vi "Power Values (Multiple Lines).vi"(0 "phase voltage spectra":T2(array[cluster]), 5 "current spectra":T2(array[cluster]), 9 "system info in":refnum<class "EP System Info.lvclass">, 11 "error in (no error)":errorcluster) -> (4 "power values":T4, 6 "3-phase power values":T3, 10 "system info out":refnum<class "EP System Info.lvclass">, 15 "error out":errorcluster)   [LabVIEW 2014, in "NI_EP_Power Quality.lvlib"]
doc: "Calculates the power values from the voltage and current spectra of different line configurations. You must manually select the polymorphic instance you want to use."
uses:
  <vilib>/addons/Electrical Power/PQ/NI_EP_Power Quality.lvlib
  <vilib>/addons/Electrical Power/PQ/Common/Classes/System Info/EP System Info.lvclass
  <vilib>/addons/Electrical Power/PQ/Common/Controls/ep_AI Data Channel.ctl
  <vilib>/addons/Electrical Power/Basic/NI_EP_Basic.lvlib
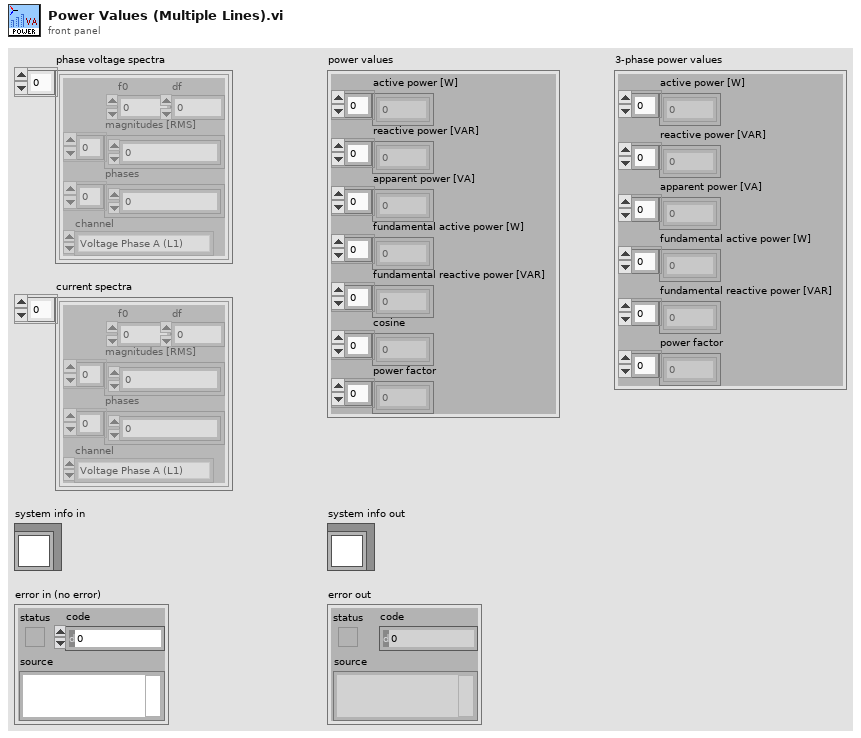
[diagram p1: front panel]
types:
  T1 = typedef "NI_EP_Power Quality.lvlib/ep_AI Data Channel.ctl" = enum16{"Voltage Phase A (L1)", "Voltage Phase B (L2)", "Voltage Phase C (L3)", "Voltage Phase N (Neutral)", "Current Phase A (L1)", "Current Phase B (L2)", "Current Phase C (L3)", "Current Phase N (Neutral)"}
  T2 = cluster{"f0":dbl, "df":dbl, "magnitudes [RMS]":dbl[], "phases":dbl[], "channel":T1}[]
  T3 = cluster{"active power [W]":dbl[], "reactive power [VAR]":dbl[], "apparent power [VA]":dbl[], "fundamental active power [W]":dbl[], "fundamental reactive power [VAR]":dbl[], "power factor":dbl[]}
  T4 = cluster{"active power [W]":dbl[], "reactive power [VAR]":dbl[], "apparent power [VA]":dbl[], "fundamental active power [W]":dbl[], "fundamental reactive power [VAR]":dbl[], "cosine":dbl[], "power factor":dbl[]}
  T5 = cluster{"active power P (W)":dbl[], "reactive power Q (VAr)":dbl[], "apparent power S (VA)":dbl[], "fundamental active power P1 (W)":dbl[], "fundamental reactive power Q1 (VAr)":dbl[], "cosine":dbl[], "power factor PF":dbl[]}
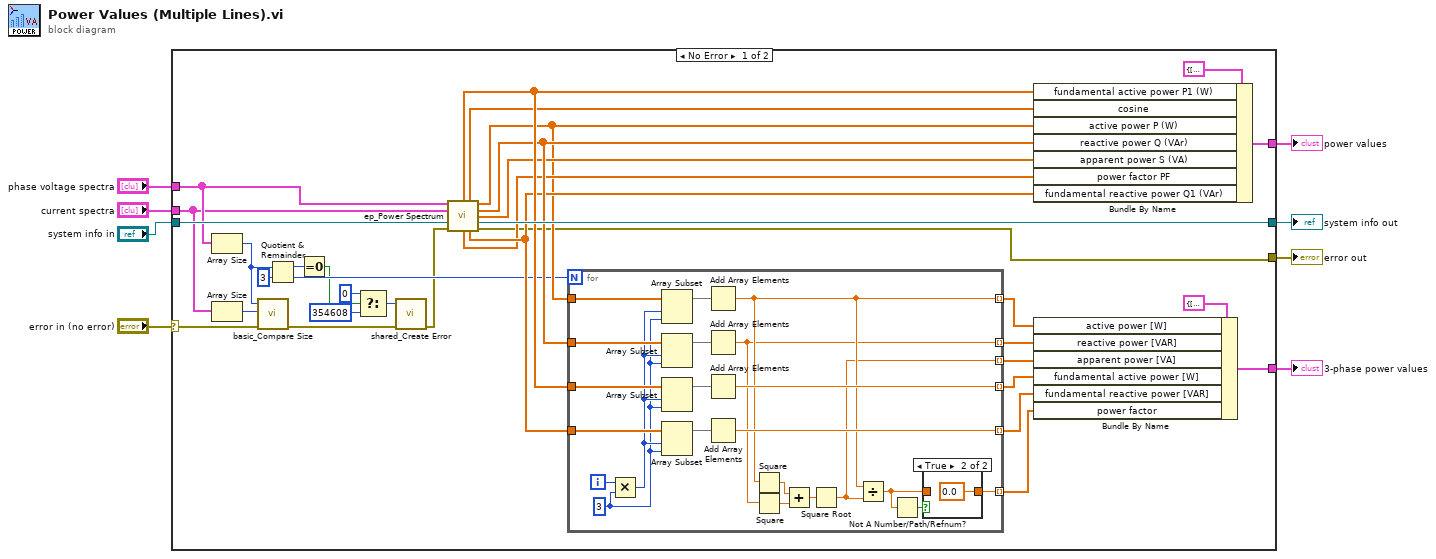
[diagram p0: block diagram]
diagram:
  n1 = case shown="No Error" "error in (no error)" {
    selector: "error in (no error)" -> [w20 w68]
    tunnel: [w42 _] -> w6
    tunnel: [w40 _] -> w7
    tunnel: "system info in" -> [w36 w67]
    tunnel: "current spectra" -> [w18 _]
    tunnel: "phase voltage spectra" -> [w19 _]
    tunnel: [w35 w67] -> w8
    tunnel: [w9 w68] -> w5
    frame No Error {
      n2 = Array Size(array=w19) -> (size(s)=w17:i32)
      n3 = Array Size(array=w18) -> (size(s)=w21:i32)
      n4 = call <vilib>:"basic_Compare Size.vi"("error in (no error)"=w20, "size B"=w21, "size A"=w17) -> ("error out"=w13:errorcluster)  [unwired: 8 in]
      n5 = Quotient & Remainder(x=w17, y=3) -> (x-y*floor(x/y)=w12:i32, floor(x/y)=w22:i32)
      n6 = Equal To 0?(x=w12) -> (x = 0?=w11:bool)
      n7 = Select(t=0, s=w11, f=354608) -> (s? t:f=w14:i32)
      n8 = call <vilib>:"shared_Create Error.vi"("error in (no error)"=w13, "error code (0)"=w14) -> ("error out"=w10:errorcluster)  [unwired: 9 in]
      n9 = call <vilib>:"ep_Power Spectrum.vi"("phase voltage spectra (5Hz step)"=w19, "current spectra (5Hz step)"=w18, "system info in"=w36, "error in (no error)"=w10) -> ("fundamental active power P1 (W)"=w34:dbl[], "cosine"=w33:dbl[], "active power P (W)"=w24:dbl[], "reactive power Q (VAr)"=w32:dbl[], "apparent power S (VA)"=w31:dbl[], "system info out"=w35:refnum<class "EP System Info.lvclass">, "power factor PF"=w29:dbl[], "fundamental reactive power Q1 (VAr)"=w30:dbl[], "error out"=w9:errorcluster)  [unwired: 3 in]
      n10 = for {
        N: w22 -> [_]
        tunnel: [w64] -> w39 mode=indexing
        tunnel: [w63] -> w38 mode=indexing
        tunnel: [w60] -> w37 mode=indexing
        tunnel: w34 -> [w59]
        tunnel: w24 -> [w58]
        tunnel: w32 -> [w57]
        tunnel: w30 -> [w56]
        tunnel: [w55] -> w28 mode=indexing
        tunnel: [w54] -> w27 mode=indexing
        tunnel: [w50] -> w26 mode=indexing
        i -> [w48]
        w43 = 3 ("y")
        n11 = Multiply(x=w48, y=w43) -> (x*y=w44:i32)
        n12 = Array Subset(array=w58, index=w44, length=w43) -> (w49:dbl[])
        n13 = Array Subset(array=w57, index=w44, length=w43) -> (w47:dbl[])
        n14 = Array Subset(array=w59, index=w44, length=w43) -> (w46:dbl[])
        n15 = Array Subset(array=w56, index=w44, length=w43) -> (w45:dbl[])
        n16 = Add Array Elements(numeric array=w49) -> (sum=w55:dbl)
        n17 = Add Array Elements(numeric array=w47) -> (sum=w54:dbl)
        n18 = Add Array Elements(numeric array=w46) -> (sum=w64:dbl)
        n19 = Add Array Elements(numeric array=w45) -> (sum=w63:dbl)
        n20 = Square(x=w55) -> (x^2=w53:dbl)
        n21 = Square(x=w54) -> (x^2=w52:dbl)
        n22 = Add(x=w53, y=w52) -> (x+y=w51:dbl)
        n23 = Square Root(x=w51) -> (sqrt(x)=w50:dbl)
        n24 = Divide(x=w55, y=w50) -> (x/y=w62:dbl)
        n25 = Not A Number/Path/Refnum?(number/path/refnum=w62) -> (NaN/Path/Refnum?=w61:bool)
        n26 = case shown="True" w61 {
          tunnel: w62 -> [w65 _]
          tunnel: [w65 0.0] -> w60
          frame False {
          }
          frame True {
          }
        }
      }
      n27 = Bundle By Name(cluster=T5 {"active power P (W)"=[], "reactive power Q (VAr)"=[], "apparent power S (VA)"=[], "fundamental active power P1 (W)"=[], "fundamental reactive power Q1 (VAr)"=[], "cosine"=[], "power factor PF"=[]} ("power values"), "fundamental active power P1 (W)"=w34, "cosine"=w33, "active power P (W)"=w24, "reactive power Q (VAr)"=w32, "apparent power S (VA)"=w31, "power factor PF"=w29, "fundamental reactive power Q1 (VAr)"=w30) -> (w42:T5)
      n28 = Bundle By Name(cluster=T3 {"active power [W]"=[], "reactive power [VAR]"=[], "apparent power [VA]"=[], "fundamental active power [W]"=[], "fundamental reactive power [VAR]"=[], "power factor"=[]} ("3-phase power values"), "active power [W]"=w28, "reactive power [VAR]"=w27, "apparent power [VA]"=w26, "fundamental active power [W]"=w39, "fundamental reactive power [VAR]"=w38, "power factor"=w37) -> (w40:T3)
    }
    frame Error {
    }
  }
  "error out" <- w5
  "power values" <- w6
  "system info out" <- w8
  "3-phase power values" <- w7
